vi "数据流模式.vi"() -> ()   [LabVIEW 2013]
panel:
  out "x/y":dbl
  in  "数值 2":dbl
  in  "数值":dbl
  out "数组":dbl[](array[numeric])
  out "number: 0 to 1":dbl
  in  "停止":bool
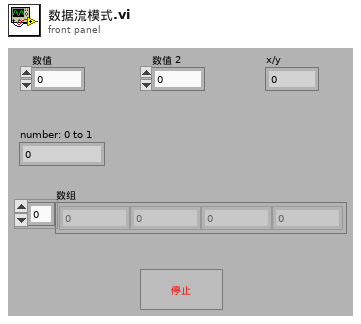
[diagram p1: front panel]
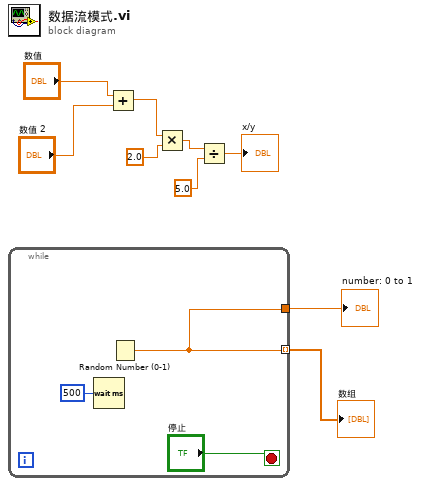
[diagram p0: block diagram]
diagram:
  n1 = while {
    tunnel: [w11] -> w9 mode=indexing
    tunnel: [w11] -> w8
    stop <- "停止" stop-if-true
    n2 = Wait (ms)(milliseconds to wait=u32 500 ("等待时间（毫秒）")) -> ()  [unwired: 1 out]
    n3 = Random Number (0-1)() -> (number: 0 to 1=w11:dbl)
  }
  "number: 0 to 1" <- w8
  "数组" <- w9
  n4 = Add(x="数值", y="数值 2") -> (x+y=w5:dbl)
  n5 = Multiply(x=w5, y=2.0) -> (x*y=w3:dbl)
  n6 = Divide(x=w3, y=5.0) -> (x/y=→"x/y":dbl)
